vi "Read Port Output Level (Scan).vi"(8 "error in (no error)":errorcluster, 10 "Port (1)":T1=enum."1", 11 "VISA resource name":refnum<visa-resource-name>) -> (0 "error out":errorcluster, 1 "Port Output Level":dbl format="%.3g", 3 "VISA resource name out":refnum<visa-resource-name>)   [LabVIEW 2013, in "SRS SR400.lvlib"]
doc: "<B>PZ i</B>\n\nThe PZ command returns the level of the PORT1 and PORT2 outputs during a scan. i=1 or 2 to select PORT1 or PORT 2 and is required. If the selected port is in the SCAN mode, its current level during a scan is read. If the counters are in reset or the output is in the FIXED mode, the PZ command returns the starting value for the level (same as PL command). The PZ command is a read only command."
uses:
  <instrlib>/SRS SR400/SRS SR400.lvlib
  <instrlib>/SRS SR400/Public/Typedefs/Port.ctl
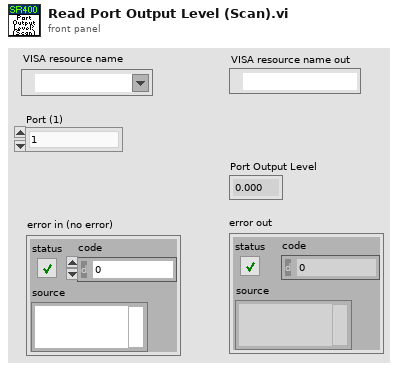
[diagram p1: front panel]
types:
  T1 = typedef "SRS SR400.lvlib/Port.ctl" = enum16{"(not used)", "1", "2"}
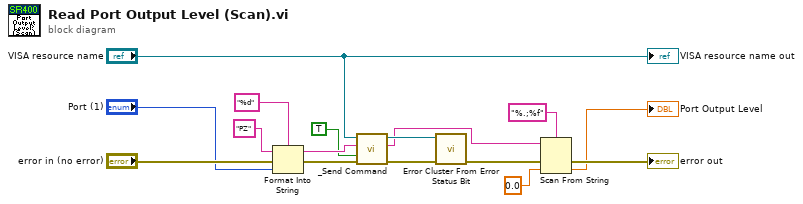
[diagram p0: block diagram]
diagram:
  n1 = Format Into String(format string="%d", initial string="PZ" ("command"), error in="error in (no error)", "Port (1)") -> (resulting string=w9:string, error out=w8:errorcluster)
  n2 = call <instrlib>:"_Send Command.vi"("error in (no error)"=w8, "Read Value? (F)"=TRUE, "Command"=w9, "VISA resource name"="VISA resource name") -> ("error out"=w4:errorcluster, "Response"=w2:string, "VISA resource name out"=w5:refnum<visa-resource-name>)  [unwired: 5 out]
  n3 = call <instrlib>:"Error Cluster From Error Status Bit.vi"("error in (no error)"=w4, "VISA resource name"=w5) -> ("error out"=w3:errorcluster)  [unwired: 8 in, 1 out]
  n4 = Scan From String(format string="%.;%f", input string=w2, error in=w3, default 1=0.0 ("default value 1")) -> (error out=→"error out":errorcluster, output 1=→"Port Output Level":dbl)  [unwired: 1 in, 2 out]
  "VISA resource name out" <- "VISA resource name"
